vi "SetExposureResolution.vi"(9 "ExpRes":refnum<k24>, 10 "Exposure Resolution":refnum<vi>, 11 "ComboBox in":refnum<vi>) -> ()   [LabVIEW 2018]
uses:
  D:/SVN/PM/sdk/AppSamples/LabVIEWSamples/trunk/Release/2018/Dependencies/PVCamNET.dll
  Dependencies/PVCamNET.dll
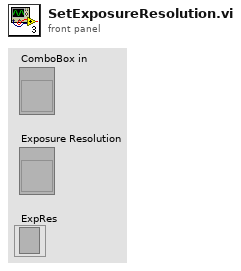
[diagram p1: front panel]
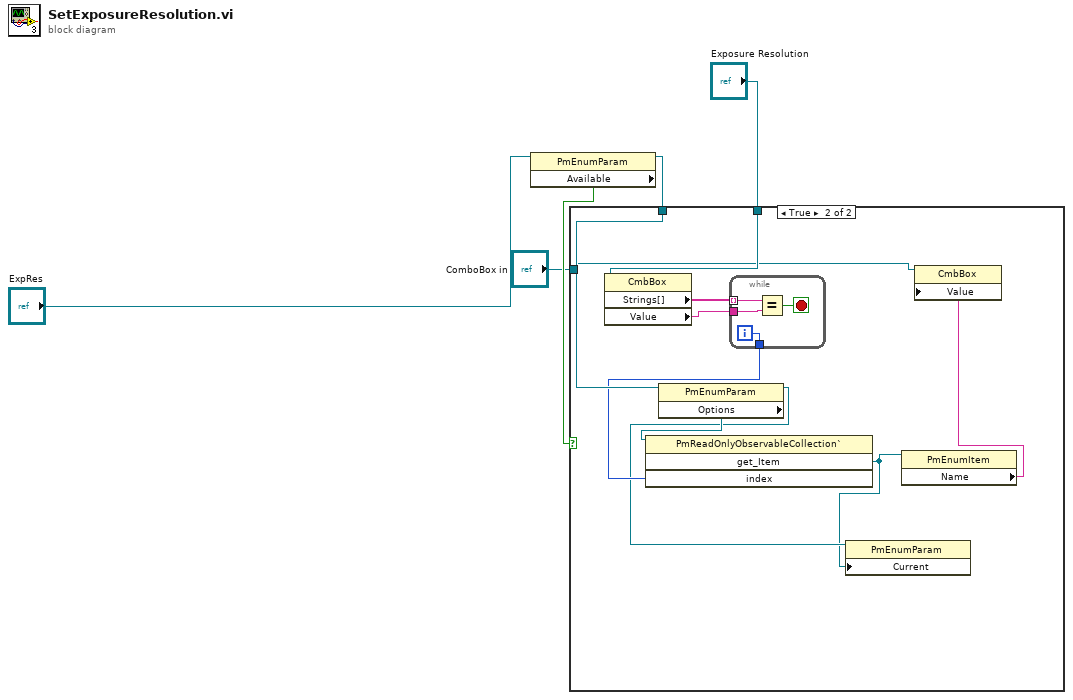
[diagram p0: block diagram]
diagram:
  n1 = property class="PmEnumParam"(reference="ExpRes") -> (reference out=w4:refnum<k24>, "Available"=w3:bool)  [unwired: 1 in, 1 out]
  n2 = case shown="True" w3 {
    tunnel: w4 -> [_ w12]
    tunnel: "Exposure Resolution" -> [_ w15]
    tunnel: "ComboBox in" -> [_ w6]
    frame False {
    }
    frame True {
      n3 = property class="CmbBox"(reference=w15) -> ("Strings[]"=w13:string[], "Value"=w14:string)  [unwired: 1 in, 2 out]
      n4 = property class="PmEnumParam"(reference=w12) -> (reference out=w9:refnum<k24>, "Options"=w11:refnum<k24>)  [unwired: 1 in, 1 out]
      n5 = while {
        tunnel: w14 -> [w19]
        tunnel: w13 -> [w18] mode=indexing
        tunnel: [w16] -> w10
        i -> [w16]
        stop <- w17 stop-if-true
        n6 = Equal?(x=w18, y=w19) -> (x = y?=w17:bool)
      }
      n7 = invoke class="PmReadOnlyObservableCollection`" method="get_Item"(reference=w11, "index"=w10) -> ("get_Item"=w8:refnum<k24>)  [unwired: 2 in, 3 out]
      n8 = property class="PmEnumParam"(reference=w9, "Current"=w8) -> ()  [unwired: 1 in, 2 out]
      n9 = property class="PmEnumItem"(reference=w8) -> ("Name"=w7:string)  [unwired: 1 in, 2 out]
      n10 = property class="CmbBox"(reference=w6, "Value"=w7) -> ()  [unwired: 1 in, 2 out]
    }
  }
